vi "module.vi"(6 "cmd channel":T1) -> (7 "response":T1)   [LabVIEW 2023]
uses:
  <vilib>/DLR/CMH Lib/Message Queue.lvlib
  <vilib>/DLR/CMH Lib/Message Queue Helper.lvlib
  <vilib>/DLR/CMH Lib/Message Queue/Enqueue Message.vi
  <extravilib>/ChannelInstances/Event Messenger-bool.lvlib
  480c1a3a-5302-4998-8e9b-bb535253195f.vi
  <vilib>/DLR/CMH Lib/Message Queue/Message Cluster.ctl
  <extravilib>/ChannelInstances/Messenger-t'Message Queue.lvlib-Message Cluster.ctl'/))Channel.ctl
  <extravilib>/ChannelInstances/Messenger-t'Message Queue.lvlib-Message Cluster.ctl'.lvlib
panel:
  in  "Main Control":enum32{"Temperature", "Series"}(tab)
  in  "Close Button":bool
  out "Log":string
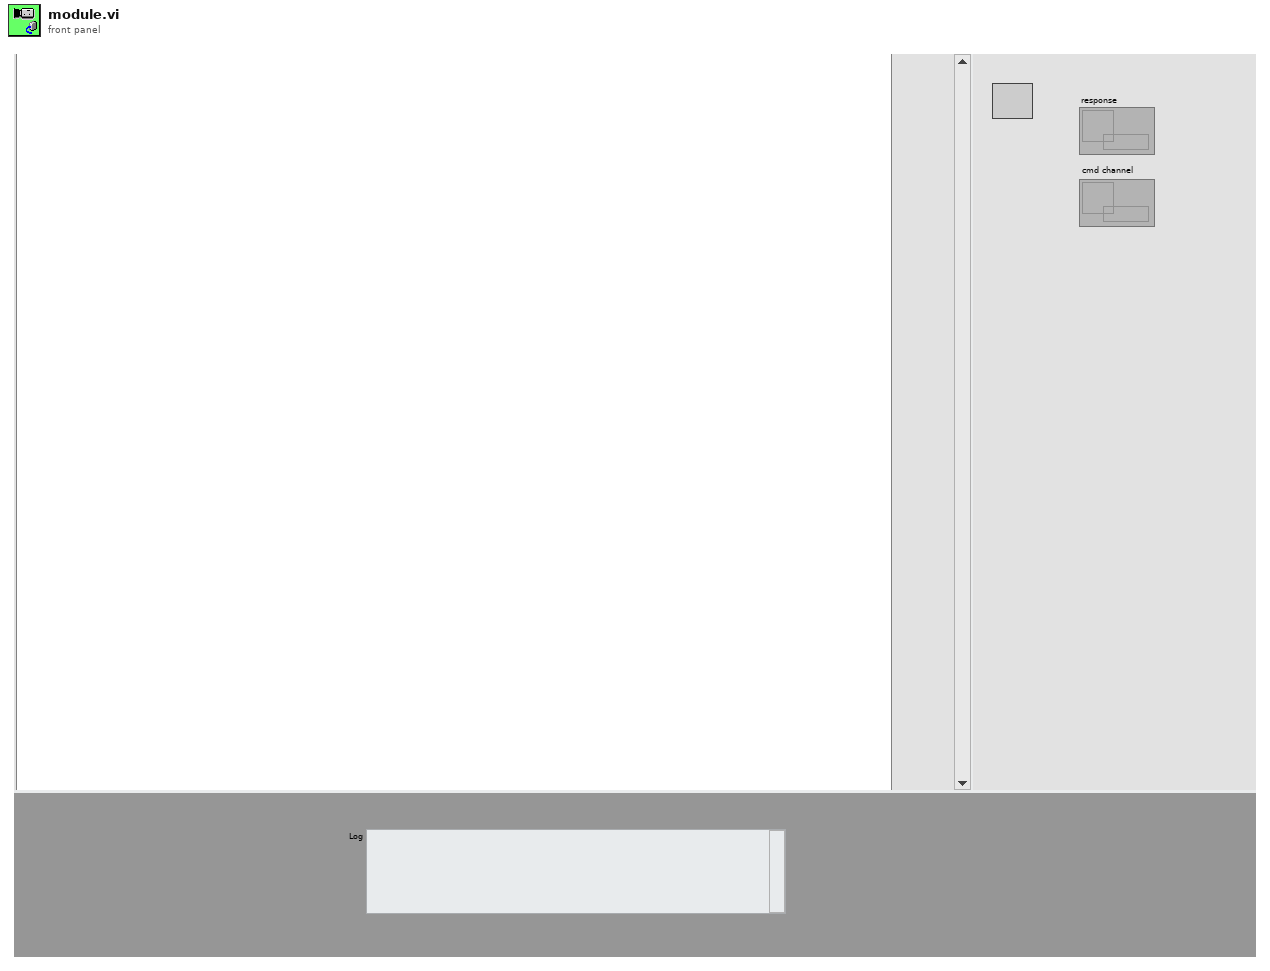
[diagram p1: front panel]
types:
  T1 = typedef "Messenger-t'Message Queue.lvlib-Message Cluster.ctl'.lvlib/))Channel.ctl" = refnum<queue>
  T2 = typedef "Event Messenger-bool.lvlib/))Channel.ctl" = refnum<queue>
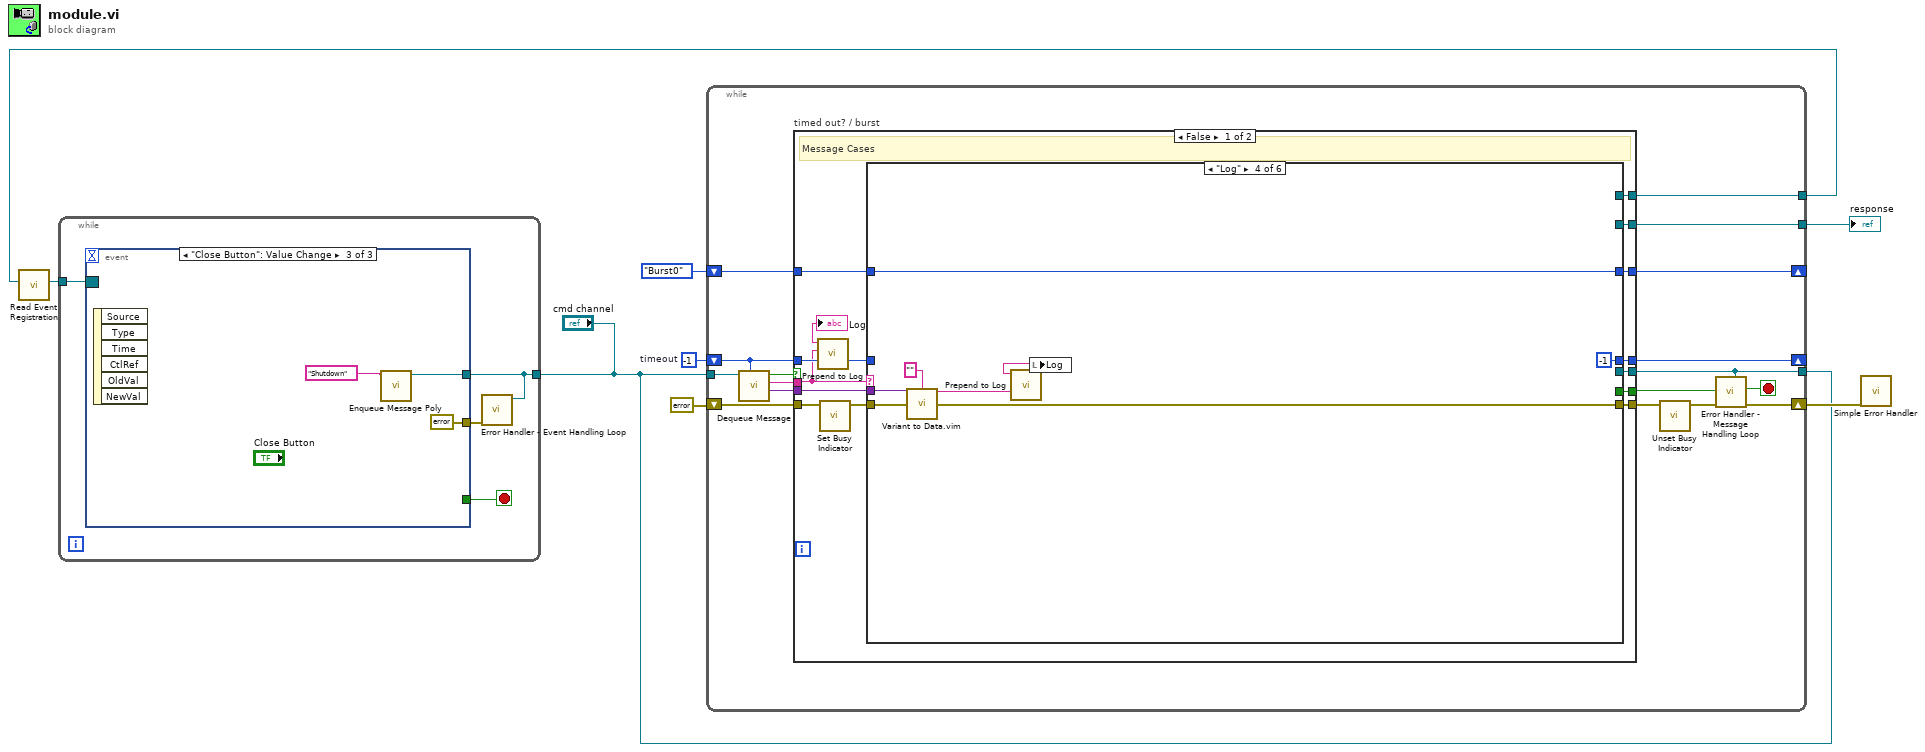
[diagram p0: block diagram]
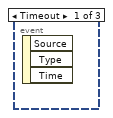
[diagram p2: hidden frame]
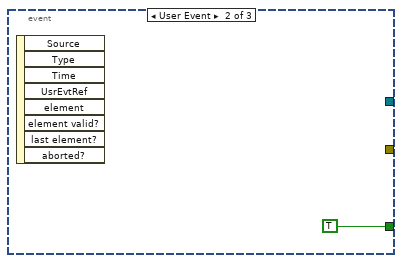
[diagram p3: hidden frame]
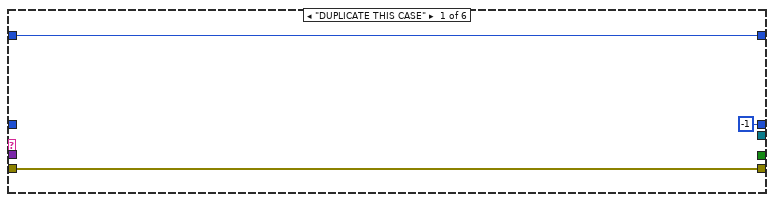
[diagram p4: hidden frame]
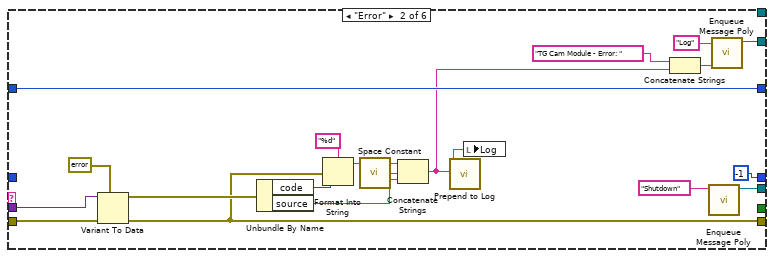
[diagram p5: hidden frame]
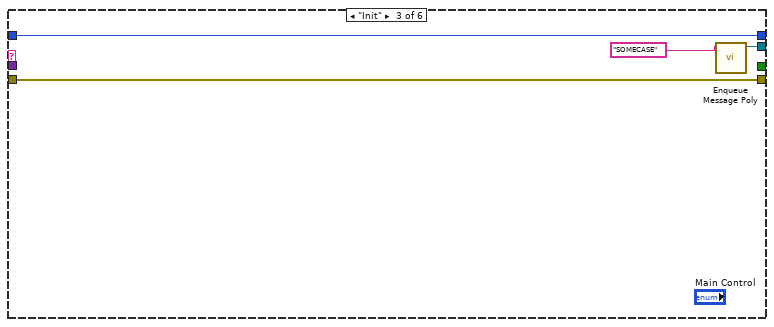
[diagram p6: hidden frame]
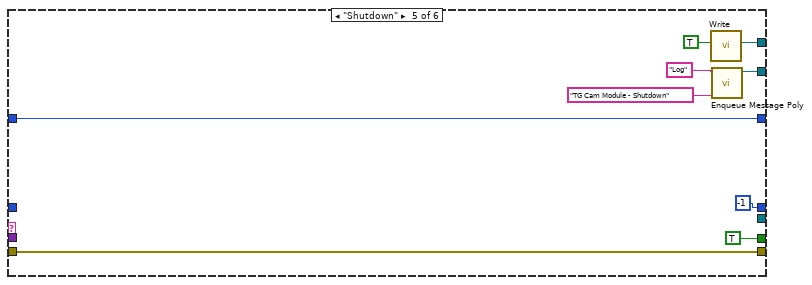
[diagram p7: hidden frame]
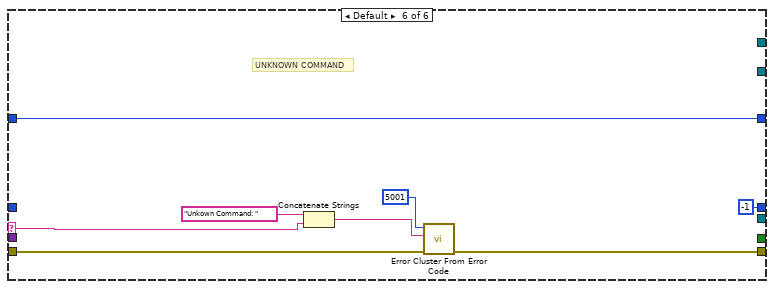
[diagram p8: hidden frame]
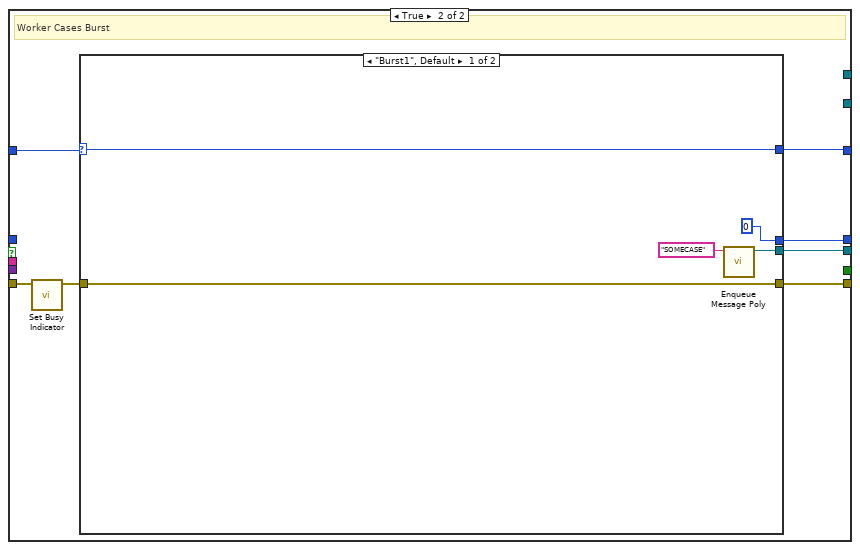
[diagram p9: hidden frame]
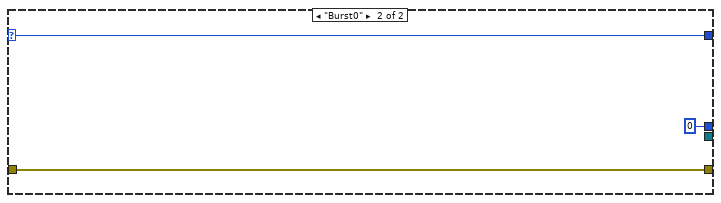
[diagram p10: hidden frame]
diagram:
  w7 = -1  # timeout
  n1 = call <extravilib>:"Read Event Registration.vi"("channel"=w5) -> ("event registration refnum"=w4:refnum<event-registration>)  [unwired: 10 in]
  n2 = while {
    tunnel: [w9] -> w1
    tunnel: w4 -> [w11]
    stop <- w12 stop-if-true
    n3 = event shown="[2] \"Close Button\": Value Change" {
      selector: w11 -> [_ _ _]
      dyn-events: _ -> [_ _ _]
      timeout: _ -> [_ _ _]
      tunnel: [_ _ w16] -> w9
      tunnel: [_ TRUE _] -> w12
      tunnel: [_ _ errorcluster {"status"=FALSE, "code"=0, "source"=""} ("error out")] -> w10
      event Timeout {
        n4 = event-data() -> ()  [unwired: 1 in, 3 out]
      }
      event User Event {
        n5 = event-data() -> ()  [unwired: 1 in, 8 out]
      }
      event "Close Button": Value Change {
        n6 = event-data() -> ()  [unwired: 1 in, 6 out]
        n7 = call-poly <vilib>:"Enqueue Message Poly.vi"("Message"="Shutdown") -> ("channel"=w16:T1)  [unwired: 10 in]
      }
    }
    n8 = call <vilib>:"Error Handler - Event Handling Loop.vi"("channel"=w9, "error in (no error)"=w10) -> ()  [unwired: 9 in, 1 out]
  }
  "cmd channel" <- w1
  n9 = while {
    tunnel: w1 -> [w33]
    shift-right: [w31] -> _
    shift-left: w7 -> [w22]
    tunnel: w1 -> [w27]
    shift-right: [w28] -> _
    shift-left: enum16{"Burst0", "Burst1"}."Burst0" -> [w29]
    tunnel: [w21] -> w5
    shift-right: [w24] -> w2
    shift-left: errorcluster {"status"=FALSE, "code"=0, "source"=""} ("error constant") -> [w18]
    tunnel: [w19] -> w3
    stop <- w25 stop-if-true
    n10 = call <vilib>:"Dequeue Message.vi"("timeout in ms (-1)"=w22, "channel"=w33) -> ("message data"=w32:variant, "message"=w20:string, "timed out?"=w23:bool)  [unwired: 7 in]
    n11 = case "timed out? / burst" shown="False" w23 {
      tunnel: w18 -> [w47 w102]
      tunnel: [w41 w100] -> w30
      tunnel: [w46 _] -> w26
      tunnel: w32 -> [w45 _]
      tunnel: w20 -> [w36 _]
      tunnel: [w44 w104] -> w31
      tunnel: w29 -> [w40 w106]
      tunnel: [w43 w105] -> w28
      tunnel: [w42 w103] -> w27
      tunnel: w22 -> [w39 _]
      tunnel: [w38 _] -> w21
      tunnel: [w35 _] -> w19
      frame False {
        # "Message Cases"
        n12 = call <vilib>:"Prepend to Log.vi"("new entry"=w36) -> ("Log out"=→"Log":string)  [unwired: 10 in]
        n13 = call <vilib>:"Set Busy Indicator.vi"("error in (no error)"=w47) -> ("error out"=w34:errorcluster)  [unwired: 10 in]
        n14 = case shown="\"Log\"" w36 {
          selector: w36 -> [_ _ _ _ _ w92]
          tunnel: w45 -> [_ w60 _ w76 _ _]
          tunnel: w34 -> [w48 w63 w73 w80 w89 w94]
          tunnel: [_ _ _ _ TRUE _] -> w46
          tunnel: [-1 ("repeat") -1 ("repeat") w71 -1 ("repeat") -1 ("repeat") -1 ("repeat")] -> w44
          tunnel: [w49 w69 _ w81 w88 w98] -> w43
          tunnel: [_ w57 w74 _ _ _] -> w42
          tunnel: [w48 w59 w73 w78 w89 w93] -> w41
          tunnel: w40 -> [w49 w69 _ w81 w88 w98]
          tunnel: w39 -> [_ _ w71 _ _ _]
          tunnel: [_ _ _ _ w86 _] -> w38
          tunnel: [_ w53 _ _ w84 _] -> w35
          frame "DUPLICATE THIS CASE" {
          }
          frame "Error" {
            n15 = Variant To Data(error in=w63, type=errorcluster {"status"=FALSE, "code"=0, "source"=""} ("error in (no error)"), Variant=w60) -> (data=w62:errorcluster, error out=w59:errorcluster)
            n16 = Unbundle By Name(w62) -> ("code"=w68:i32, "source"=w65:string)
            n17 = Format Into String(format string="%d", error in=w59, w68) -> (resulting string=w67:string)  [unwired: 1 in, 1 out]
            n18 = call <vilib>:"Space Constant.vi"() -> ("String"=w66:string)
            n19 = Concatenate Strings(w67, w66, w65) -> (w51:string)
            n20 = call <vilib>:"Prepend to Log.vi"("new entry"=w51) -> ("Log out"=w58:string)  [unwired: 10 in]
            n21 = local write "Log"(w58) -> ()
            n22 = Concatenate Strings("TG Cam Module - Error: " ("Message"), w51) -> (w52:string)
            n23 = call-poly <vilib>:"Enqueue Message Poly.vi"("Message"="Shutdown") -> ("channel"=w57:T1)  [unwired: 10 in]
            n24 = call-poly <vilib>:"Enqueue Message Poly.vi"("Message Data"=w52, "Message"="Log") -> ("channel"=w53:T1)  [unwired: 9 in]
          }
          frame "Init" {
            n25 = call-poly <vilib>:"Enqueue Message Poly.vi"("Message"="SOMECASE") -> ("channel"=w74:T1)  [unwired: 10 in]
          }
          frame "Log" {
            n26 = call "Variant to Data.vim"("variant"=w76, "type"="", "Error In"=w80) -> ("data"=w75:string, "Error Out"=w78:errorcluster)  [unwired: 11 in]
            n27 = call <vilib>:"Prepend to Log.vi"("new entry"=w75) -> ("Log out"=w79:string)  [unwired: 10 in]
            n28 = local write "Log"(w79) -> ()
          }
          frame "Shutdown" {
            n29 = call <extravilib>:"Write.vi"("element"=TRUE) -> ("channel"=w86:T2)  [unwired: 9 in, 1 out]
            n30 = call-poly <vilib>:"Enqueue Message Poly.vi"("Message Data"="TG Cam Module - Shutdown" ("Message"), "Message"="Log") -> ("channel"=w84:T1)  [unwired: 9 in]
          }
          frame Default {
            # "UNKNOWN COMMAND"
            n31 = Concatenate Strings("Unkown Command: ", w92) -> (w96:string)
            n32 = call <vilib>:"Error Cluster From Error Code.vi"("error in (no error)"=w94, "error message (\"\")"=w96, "error code (0)"=5001) -> ("error out"=w93:errorcluster)  [unwired: 6 in]
          }
        }
      }
      frame True {
        # "Worker Cases Burst"
        n33 = call <vilib>:"Set Busy Indicator.vi"("error in (no error)"=w102) -> ("error out"=w101:errorcluster)  [unwired: 10 in]
        n34 = case shown="\"Burst1\", Default" w106 {
          selector: w106 -> [w110 w114]
          tunnel: w101 -> [w111 w113]
          tunnel: [w111 w113] -> w100
          tunnel: [w110 w114] -> w105
          tunnel: [0 ("repeat") 0 ("repeat")] -> w104
          tunnel: [w108 _] -> w103
          frame "Burst1", Default {
            n35 = call-poly <vilib>:"Enqueue Message Poly.vi"("Message"="SOMECASE") -> ("channel"=w108:T1)  [unwired: 10 in]
          }
          frame "Burst0" {
          }
        }
      }
    }
    n36 = call <vilib>:"Unset Busy Indicator.vi"("error in (no error)"=w30) -> ("error out"=w17:errorcluster)  [unwired: 10 in]
    n37 = call <vilib>:"Error Handler - Message Handling Loop.vi"("channel"=w27, "error in (no error)"=w17, "Shutdown?"=w26) -> ("dup error in"=w24:errorcluster, "Shutdown!"=w25:bool)  [unwired: 7 in]
  }
  "response" <- w3
  n38 = call <vilib>:"Simple Error Handler.vi"("error in (no error)"=w2) -> ()  [unwired: 4 in, 5 out]
